vi "Add Monitoring Channels.vi"(8 "error in (no error)":errorcluster, 9 "progress queue":refnum<queue>, 10 "Framework Configuration":refnum<class "Framework Configuration.lvclass">=refnum, 11 "Item Ref in":T1 format="%.0x") -> (0 "error out":errorcluster, 3 "Item Ref out":T1 format="%.0x")   [LabVIEW 2019, in "DSF System Explorer.lvlib"]
uses:
  DSF System Explorer.lvlib
  <vilib>/NI VeriStand/Custom Device API/Custom Device Channel Type.ctl
  <vilib>/NI VeriStand/Custom Device API/Custom Device API.lvlib
  <vilib>/NI VeriStand/Custom Device API/Custom Device Channel.ctl
  Shared/DSF Shared.lvlib
  <vilib>/NI VeriStand/Custom Device API/Custom Device Item Ref.ctl
  DSF Core.lvlibp/Classes/Configuration/Core/Framework/Framework Configuration.lvclass
  progress window data.ctl
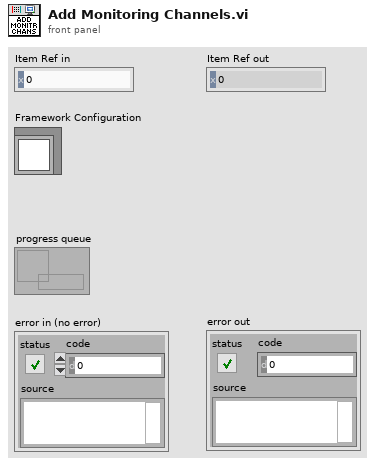
[diagram p1: front panel]
types:
  T1 = typedef "Custom Device API.lvlib/Custom Device Item Ref.ctl" = u64
  T2 = typedef "Custom Device API.lvlib/Custom Device Channel.ctl" = cluster{"Type":T3, "Units":string, "Default Value":dbl, "Faultable":bool, "Scalable":bool}
  T3 = typedef "Custom Device API.lvlib/Custom Device Channel Type.ctl" = enum16{"Input", "Output"}
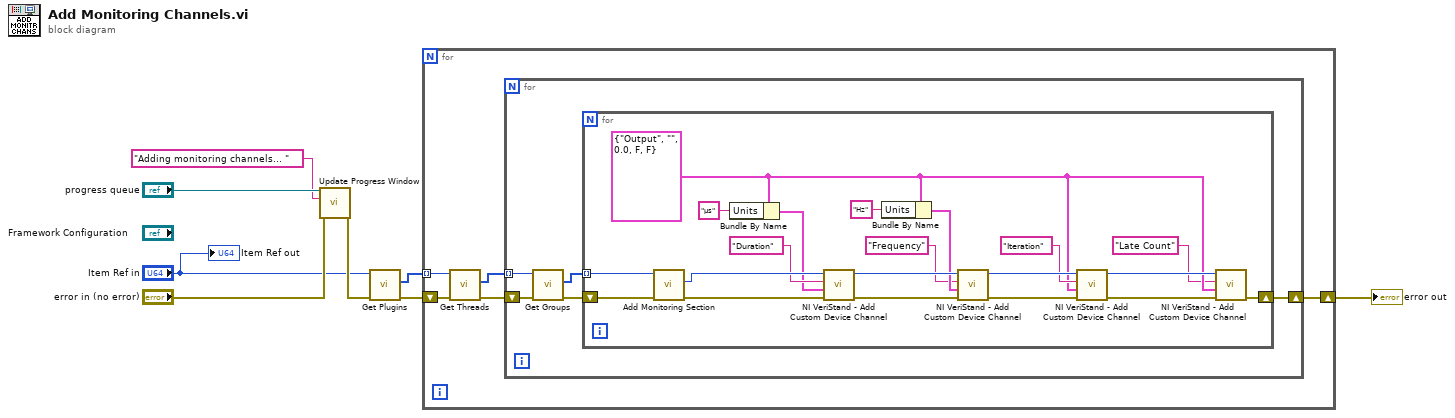
[diagram p0: block diagram]
diagram:
  n1 = call "Update Progress Window.vi"("error in (no error)"="error in (no error)", "message (\"\")"="Adding monitoring channels... " ("message (\"\")"), "progress queue in"="progress queue") -> ("error out"=w4:errorcluster)  [unwired: 7 in, 1 out]
  n2 = call "Get Plugins.vi"("error in (no error)"=w4, "Item Ref in"="Item Ref in") -> ("error out"=w3:errorcluster, "Plugin refs"=w1:T1[])  [unwired: 7 in, 1 out]
  n3 = for {
    tunnel: w1 -> [w11] mode=indexing
    shift-right: [w13] -> w5
    shift-left: w3 -> [w12]
    n4 = call "Get Threads.vi"("error in (no error)"=w12, "Item Ref in"=w11) -> ("error out"=w10:errorcluster, "Plugin refs"=w9:T1[])  [unwired: 7 in, 1 out]
    n5 = for {
      tunnel: w9 -> [w16] mode=indexing
      shift-right: [w18] -> w13
      shift-left: w10 -> [w17]
      n6 = call "Get Groups.vi"("error in (no error)"=w17, "Plugin Ref in"=w16) -> ("error out"=w15:errorcluster, "Group refs"=w14:T1[])  [unwired: 7 in, 1 out]
      n7 = for {
        tunnel: w14 -> [w23] mode=indexing
        shift-right: [w36] -> w18
        shift-left: w15 -> [w24]
        w26 = T2 {"Type"=enum."Output", "Units"="", "Default Value"=0.0, "Faultable"=FALSE, "Scalable"=FALSE} ("Channel")
        n8 = call "Add Monitoring Section.vi"("error in (no error)"=w24, "Item Ref in"=w23) -> ("error out"=w22:errorcluster, "Performance Section Ptr"=w21:T1)  [unwired: 7 in, 1 out]
        n9 = Bundle By Name(cluster=w26, "Units"="µs" ("Section Name")) -> (w19:T2)
        n10 = call <vilib>:"NI VeriStand - Add Custom Device Channel.vi"("error in (no error)"=w22, "Channel"=w19, "Channel Name"="Duration" ("Section Name"), "Parent Ref in"=w21) -> ("error out"=w35:errorcluster, "Parent Ref out"=w34:T1)  [unwired: 4 in, 2 out]
        n11 = Bundle By Name(cluster=w26, "Units"="Hz") -> (w29:T2)
        n12 = call <vilib>:"NI VeriStand - Add Custom Device Channel.vi"("error in (no error)"=w35, "Channel"=w29, "Channel Name"="Frequency" ("Section Name"), "Parent Ref in"=w34) -> ("error out"=w33:errorcluster, "Parent Ref out"=w32:T1)  [unwired: 4 in, 2 out]
        n13 = call <vilib>:"NI VeriStand - Add Custom Device Channel.vi"("error in (no error)"=w33, "Channel"=w26, "Channel Name"="Iteration" ("Section Name"), "Parent Ref in"=w32) -> ("error out"=w31:errorcluster, "Parent Ref out"=w30:T1)  [unwired: 4 in, 2 out]
        n14 = call <vilib>:"NI VeriStand - Add Custom Device Channel.vi"("error in (no error)"=w31, "Channel"=w26, "Channel Name"="Late Count" ("Section Name"), "Parent Ref in"=w30) -> ("error out"=w36:errorcluster)  [unwired: 4 in, 3 out]
      }
    }
  }
  "error out" <- w5
  "Item Ref out" <- "Item Ref in"
